vi "BonOMM-SAOMM.vi"() -> ()   [LabVIEW 2019] (continued)
                                n1515 = Bundle(w5154, w5153, "X"=w5137, "Y"=w5136) -> (w5155:cluster{void, void, "X":i32, "Y":i32})  [unwired: 1 in]
                                n1516 = property class="GraphInt (strict)"(reference=w5148, "Active Cursor"=u32 0) -> ("Y Scale.Range:Maximum"=w5139:dbl, "Y Scale.Range:Minimum"=w5138:dbl, "X Scale.Range:Maximum"=w5150:dbl, "X Scale.Range:Minimum"=w5149:dbl)  [unwired: 1 in, 2 out]
                                n1517 = call "BoxCrossPict.vi"("rect"=w5155) -> ("Pict Out"=→"Picture":picture)  [unwired: 1 in, 2 out]
                                n1518 = control-ref of="Picture"() -> (w5146:refnum<vi>)
                                n1519 = property class="Image"(reference=w5146) -> ("Draw Area Size"=w5147:T40)  [unwired: 1 in, 2 out]
                                n1520 = Unbundle(w5147) -> ("Width"=w5143:u32, "Height"=w5142:u32)
                                n1521 = Subtract(x=w5142, y=u32 6) -> (x-y=w5144:u32)
                                n1522 = Subtract(x=w5143, y=u32 6) -> (x-y=w5145:u32)
                                n1523 = call "Pict_to_Graph.vi"("Xo"=w5137, "Width"=w5145, "Yo"=w5136, "Heigth"=w5144, "X Scale.Range:Minimum"=w5149, "X Scale.Range:Maximum"=w5150, "Y Scale.Range:Minimum"=w5138, "Y Scale.Range:Maximum"=w5139) -> ()  [unwired: 2 in, 2 out]
                                }
                                frame True {
                                n1524 = property class="GraphInt (strict)"(reference=w5174, "Active Cursor"=u32 0) -> (reference out=w5166:refnum<vi>, "Y Scale.Range:Maximum"=w5170:dbl, "Y Scale.Range:Minimum"=w5169:dbl, "X Scale.Range:Maximum"=w5168:dbl, "X Scale.Range:Minimum"=w5167:dbl)  [unwired: 1 in, 1 out]
                                n1525 = control-ref of="Picture"() -> (w5163:refnum<vi>)
                                n1526 = property class="Image"(reference=w5163) -> ("Draw Area Size"=w5164:T40)  [unwired: 1 in, 2 out]
                                n1527 = Unbundle(w5164) -> ("Width"=w5162:u32, "Height"=w5161:u32)
                                n1528 = Subtract(x=w5161, y=u32 6) -> (x-y=w5157:u32)
                                n1529 = Subtract(x=w5162, y=u32 6) -> (x-y=w5158:u32)
                                n1530 = call "Pict_to_Graph.vi"("Xo"=w5175, "Width"=w5158, "Yo"=w5156, "Heigth"=w5157, "X Scale.Range:Minimum"=w5167, "X Scale.Range:Maximum"=w5168, "Y Scale.Range:Minimum"=w5169, "Y Scale.Range:Maximum"=w5170) -> ("CursorY"=w5172:dbl, "CursorX"=w5173:dbl)  [unwired: 2 in]
                                n1531 = property class="GraphInt (strict)"(reference=w5166, "Active Cursor"=u32 0, "Cursor.Cursor Position:Cursor X"=w5173, "Cursor.Cursor Position:Cursor Y"=w5172) -> ()  [unwired: 1 in, 2 out]
                                }
                                }
                              }
                            }
                            frame #1 {
                              n1532 = local read item#-1() -> (w5191)
                              n1533 = local read item#-1() -> (w5188)
                              n1534 = Max & Min(x=w5191, y=w5187) -> (min(x,y)=w5185:i32)  [unwired: 1 out]
                              n1535 = Max & Min(x=w5186, y=w5188) -> (max(x,y)=w5176:i32)  [unwired: 1 out]
                              n1536 = control-ref of="ImgArray"() -> (w5177:refnum<vi>)
                              n1537 = Subtract(x=w5191, y=w5187) -> (x-y=w5189:i32)
                              n1538 = Subtract(x=w5186, y=w5188) -> (x-y=w5190:i32)
                              n1539 = control-ref of="Picture"() -> (w5178:refnum<vi>)
                              n1540 = Absolute Value(x=w5189) -> (abs(x)=w5184:i32)
                              n1541 = Absolute Value(x=w5190) -> (abs(x)=w5183:i32)
                              n1542 = call "PICT_to_CAM.vi"("Pict Refnum"=w5178, "IntGraph Refnum"=w5177, "Ny"=w5183, "Yo"=w5176, "Nx"=w5184, "Xo"=w5185) -> ("Ny CAM"=→"Naxis2":i16, "Nx CAM"=→"Naxis1":i16, "Yo CAM"=w5181:i16, "Xo CAM"=w5182:i16)
                            }
                          }
                        }
                      }
                      n1543 = Not Equal?(x=w5115, y=w5117) -> (x != y?=w5118:bool)
                      n1544 = Not Equal?(x=w5117, y=w5114) -> (x != y?=w5119:bool)
                      n1545 = And(x=w5118, y=w5119) -> (x .and. y?=w5116:bool)
                    }
                  }
                  frame Enabled {
                  }
                }
              }
              event "TableXYPos": Cursor Grab {
                n1546 = event-data() -> ("CursIdx"=w5193:i32)  [unwired: 1 in, 7 out]
                n1547 = stacked-sequence {
                  tunnel: w5193 -> [w5194 _ _]
                  frame #0 {
                    n1548 = property on="TableXYPos" class="GraphXY (strict)"("Active Cursor"=w5194) -> ()  [unwired: 2 in, 2 out]
                    n1549 = case shown="1" w5194 {
                      tunnel: [TRUE FALSE] -> w5196
                      tunnel: [FALSE TRUE] -> w5195
                      frame 1 {
                      }
                      frame 0, Default {
                      }
                    }
                    n1550 = local write "act_cible"(w5195) -> ()
                    n1551 = local write "act_sonde"(w5196) -> ()
                  }
                  frame #1 {
                    n1552 = local read "ImgData"() -> (w5201:sgl[][])
                    n1553 = while {
                      tunnel: w5201 -> [w5204]
                      stop <- w5202 stop-if-true
                      n1554 = event shown="[0] Timeout" {
                        selector: _ -> [_ _]
                        dyn-events: _ -> [_ _]
                        timeout: 100 -> [_ _]
                        tunnel: w5204 -> [_ _]
                        tunnel: [FALSE TRUE] -> w5202
                        event Timeout {
                          w5205 = u16 1 items=["Region d'intérêt", "Prévisualisation"] ("ImageUsage")
                          n1555 = event-data() -> ()  [unwired: 1 in, 2 out]
                          n1556 = property on="TableXYPos" class="GraphXY (strict)"("Active Cursor"=u32 0) -> (error out=w5209:errorcluster)  [unwired: 2 in, 1 out]
                          n1557 = property on="TableXYPos" class="GraphXY (strict)"(error in=w5209) -> ("Cursor.Cursor X"=w5217:dbl, "Cursor.Cursor Y"=w5216:dbl)  [unwired: 1 in, 2 out]
                          n1558 = local read "FieldAstrom"() -> (w5211:T4)
                          n1559 = call "xy2ad.vi"("Y (px)"=w5216, "X (px)"=w5217, "Astrometry"=w5211) -> ("DEC (°)"=w5213:dbl, "RA (°)"=w5214:dbl, "DEC (HH:MM:SS)"=w5215:dbl, "RA (HH:MM:SS.S)"=w5212:dbl)  [unwired: 5 in]
                          n1560 = local read "ImgAstrom"() -> (w5225:T4)
                          n1561 = local write "RA Cible"(w5212) -> ()
                          n1562 = local write "Dec Cible"(w5215) -> ()
                          n1563 = local read "ImgData"() -> (w5218:sgl[][])
                          n1564 = call "ad2xy.vi"("DEC"=w5213, "RA"=w5214, "Astrometry"=w5225) -> ("Y"=w5224:dbl, "X"=w5223:dbl)  [unwired: 6 in, 1 out]
                          n1565 = To Long Integer(number=w5223) -> (32bit integer=w5220:i32)
                          n1566 = To Long Integer(number=w5224) -> (32bit integer=w5219:i32)
                          n1567 = call "subimage.vi"("Ysz/2"=100 ("Xsz/2"), "Xsz/2"=100, "Yc"=w5219, "Xc"=w5220, "ImgData"=w5218) -> ("SubImg"=w5207:sgl[][])  [unwired: 6 in]
                          n1568 = Array Max & Min(array=w5207) -> (max value=w5206:sgl)  [unwired: 3 out]
                          n1569 = call "Draw_crosshair.vi"("Image IN"=w5207, "White Value"=w5206) -> ("Image OUT"=→"subimg":sgl[][])  [unwired: 13 in]
                          n1570 = local write "ImageUsage"(w5205) -> ()
                        }
                        event "TableXYPos": Cursor Release {
                          n1571 = event-data() -> ()  [unwired: 1 in, 8 out]
                        }
                      }
                    }
                  }
                  frame #2 {
                    n1572 = local write "CursorGrab"(FALSE ("CursorGrab")) -> ()
                  }
                }
                "CursorGrab" <- TRUE ("CursorGrab")
              }
              event "RA Cible", "Dec Cible", "RA Sonde", "Dec Sonde", "act_cible", "act_sonde": Mouse Down {
                n1573 = event-data() -> ("CtlRef"=w5232:refnum<vi>)  [unwired: 1 in, 6 out]
                n1574 = property class="Cmde"(reference=w5232) -> ("Label.Text"=w5231:string)  [unwired: 1 in, 2 out]
                n1575 = case shown="\"Dec Cible\", \"RA Cible\", \"act_cible\", Par défaut" w5231 {
                  tunnel: [TRUE FALSE] -> w5229
                  tunnel: [FALSE TRUE] -> w5230
                  frame "Dec Sonde", "RA Sonde", "act_sonde" {
                  }
                  frame "Dec Cible", "RA Cible", "act_cible", Default {
                  }
                }
                "act_sonde" <- w5229
                "act_cible" <- w5230
              }
              event "N.O. A.D.", "N.O. Déc.", "NO epoch": Value Change {
                # "Peut-être qu'ici on"
                n1576 = event-data() -> ()  [unwired: 1 in, 6 out]
                n1577 = local read "N.O. Déc."() -> (w5250:string)
                n1578 = local read "N.O. A.D."() -> (w5251:string)
                n1579 = call "format_coords_str(new).vi"("DEC str"=w5250, "RA str"=w5251) -> ("%s DEC"=w5248:string, "%s RA"=w5249:string)  [unwired: 1 in]
                n1580 = local read "NO epoch"() -> (w5247:dbl)
                n1581 = call "time-str-to-time-dbl-RA.vi"("Chaîne"=w5249) -> ("TCS_coords"=w5240:dbl)
                n1582 = call "time-str-to-time-dbl-DEC.vi"("Chaîne"=w5248) -> ("TCS_coords"=w5238:dbl)
                n1583 = local read "LST"() -> (w5246:dbl)
                n1584 = expression code="x*3600"(w5240) -> (w5239:dbl)
                n1585 = expression code="x*3600"(w5238) -> (w5237:dbl)
                n1586 = call "Object_properties.vi"("Target RA"=w5239, "Target DEC"=w5237, "Target Epoch"=w5247, "Sideral Time"=w5246) -> ("NO RA"=w5245:string, "NO DEC"=w5244:string, "NO Epoch"=w5242:dbl, "NO HA"=w5241:dbl, "NO AM"=w5243:dbl)  [unwired: 7 in]
                n1587 = local write "NO AM"(w5243) -> ()
                n1588 = local write "NO HA"(w5241) -> ()
                n1589 = local write "NO epoch"(w5242) -> ()
                n1590 = local write "N.O. Déc."(w5244) -> ()
                n1591 = local write "N.O. A.D."(w5245) -> ()
              }
              event "Flat": Value Change {
                n1592 = event-data() -> ("NewVal"=w5255:bool)  [unwired: 1 in, 4 out]
                n1593 = Select(t="Ouverture" ("Indicateur d'état"), s=w5255, f="Fermeture" ("Indicateur d'état")) -> (s? t:f=w5259:string)
                n1594 = local read "Calib VRN"() -> (w5263:refnum<visa-resource-name>)
                n1595 = Concatenate Strings(w5259, " de la lampe de flat" ("Indicateur d'état")) -> (w5262:string)
                n1596 = control-ref of="TERMINAL"() -> (w5256:refnum<vi>)
                n1597 = control-ref of="Indicateur d'état"() -> (w5257:refnum<vi>)
                n1598 = Build Array("Arc", "Néon", w5255) -> (w5264:bool[])
                n1599 = call "Controle_des_lampe.vi"("VISA resource name"=w5263, "Status In"=w5264) -> ("Status Out"=w5254:bool[])  [unwired: 2 out]
                n1600 = local write "Status lamp"(w5254) -> ()
                n1601 = call "TERMINAL.vi"("Indicateur Refnum"=w5257, "Terminal Refnum"=w5256, "Indicateur d'état"=w5262) -> ()
                n1602 = Index Array(array=w5254, index=0 ("Index")) -> (element=→"ArcOn":bool)
                n1603 = Index Array(array=w5254, index=1 ("Index")) -> (element=→"NeonOn":bool)
                n1604 = Index Array(array=w5254, index=2 ("Index")) -> (element=→"FlatOn":bool)
                n1605 = Boolean Array To Number(Boolean array=w5254) -> (number=w5253:u32)
                n1606 = Greater Than 0?(x=w5253) -> (x > 0?=w5252:bool)
                n1607 = property on="lampOn?" class="Bool (strict)"("Blinking"=w5252, "Visible"=w5252) -> ()  [unwired: 2 in, 2 out]
              }
              event "Néon": Value Change {
                n1608 = event-data() -> ("NewVal"=w5276:bool)  [unwired: 1 in, 4 out]
                n1609 = local read "Arc"() -> (w5293:bool)
                n1610 = Select(t="Ouverture" ("Indicateur d'état"), s=w5276, f="Fermeture" ("Indicateur d'état")) -> (s? t:f=w5280:string)
                n1611 = Build Array(w5293, w5276, "Flat") -> (w5286:bool[])
                n1612 = local read "Calib VRN"() -> (w5284:refnum<visa-resource-name>)
                n1613 = Concatenate Strings(w5280, " de la lampe de Néon" ("Indicateur d'état")) -> (w5277:string)
                n1614 = call "Controle_des_lampe.vi"("VISA resource name"=w5284, "Status In"=w5286) -> ("Status Out"=w5273:bool[])  [unwired: 2 out]
                n1615 = local write "Status lamp"(w5273) -> ()
                n1616 = control-ref of="TERMINAL"() -> (w5283:refnum<vi>)
                n1617 = control-ref of="Indicateur d'état"() -> (w5282:refnum<vi>)
                n1618 = call "TERMINAL.vi"("Indicateur Refnum"=w5282, "Terminal Refnum"=w5283, "Indicateur d'état"=w5277) -> ()
                n1619 = Boolean Array To Number(Boolean array=w5273) -> (number=w5274:u32)
                n1620 = Index Array(array=w5273, index=0 ("Index")) -> (element=w5290:bool)
                n1621 = Index Array(array=w5273, index=1 ("Index")) -> (element=w5291:bool)
                n1622 = Index Array(array=w5273, index=2 ("Index")) -> (element=w5292:bool)
                n1623 = Greater Than 0?(x=w5274) -> (x > 0?=w5275:bool)
                n1624 = local write "NeonOn"(w5291) -> ()
                n1625 = local write "ArcOn"(w5290) -> ()
                n1626 = local write "FlatOn"(w5292) -> ()
                n1627 = property on="lampOn?" class="Bool (strict)"("Blinking"=w5275, "Visible"=w5275) -> ()  [unwired: 2 in, 2 out]
              }
              event "Arc": Value Change {
                n1628 = event-data() -> ("NewVal"=w5297:bool)  [unwired: 1 in, 4 out]
                n1629 = local read "Néon"() -> (w5314:bool)
                n1630 = local read "Flat"() -> (w5306:bool)
                n1631 = Select(t="Ouverture" ("Indicateur d'état"), s=w5297, f="Fermeture" ("Indicateur d'état")) -> (s? t:f=w5301:string)
                n1632 = Build Array(w5297, w5314, w5306) -> (w5307:bool[])
                n1633 = local read "Calib VRN"() -> (w5305:refnum<visa-resource-name>)
                n1634 = call "Controle_des_lampe.vi"("VISA resource name"=w5305, "Status In"=w5307) -> ("Status Out"=w5294:bool[])  [unwired: 2 out]
                n1635 = local write "Status lamp"(w5294) -> ()
                n1636 = Concatenate Strings(w5301, " de la lampe à arc" ("Indicateur d'état")) -> (w5298:string)
                n1637 = control-ref of="TERMINAL"() -> (w5304:refnum<vi>)
                n1638 = control-ref of="Indicateur d'état"() -> (w5303:refnum<vi>)
                n1639 = Index Array(array=w5294, index=0 ("Index")) -> (element=w5311:bool)
                n1640 = Index Array(array=w5294, index=1 ("Index")) -> (element=w5312:bool)
                n1641 = Index Array(array=w5294, index=2 ("Index")) -> (element=w5313:bool)
                n1642 = Boolean Array To Number(Boolean array=w5294) -> (number=w5296:u32)
                n1643 = call "TERMINAL.vi"("Indicateur Refnum"=w5303, "Terminal Refnum"=w5304, "Indicateur d'état"=w5298) -> ()
                n1644 = Greater Than 0?(x=w5296) -> (x > 0?=w5295:bool)
                n1645 = local write "NeonOn"(w5312) -> ()
                n1646 = local write "ArcOn"(w5311) -> ()
                n1647 = local write "FlatOn"(w5313) -> ()
                n1648 = property on="lampOn?" class="Bool (strict)"("Blinking"=w5295, "Visible"=w5295) -> ()  [unwired: 2 in, 2 out]
              }
              event "ModCoor": Value Change {
                n1649 = event-data() -> ("NewVal"=w5316:bool)  [unwired: 1 in, 4 out]
                n1650 = case shown="Vrai" w5316 {
                  tunnel: [FALSE w5319] -> w5315
                  frame False {
                  }
                  frame True {
                    # "Système acquisition ou\ntechnicien est prioritaire"
                    # "Epoque=0=>courante du TCS"
                    n1651 = call "time-str-to-time-dbl-DEC.vi"("Chaîne"="N.O. Déc.") -> ("TCS_coords"=w5328:dbl)
                    n1652 = call "time-str-to-time-dbl-RA.vi"("Chaîne"="N.O. A.D.") -> ("TCS_coords"=w5327:dbl)
                    n1653 = control-ref of="TERMINAL"() -> (w5335:refnum<vi>)
                    n1654 = control-ref of="Indicateur d'état"() -> (w5336:refnum<vi>)
                    n1655 = control-ref of="TCS actif"() -> (w5320:refnum<vi>)
                    n1656 = Concatenate Strings("Chargement des coordonnées : ", "N.O. A.D.", ", ", "N.O. Déc.") -> (w5330:string)
                    n1657 = local read "TCS VRN"() -> (w5325:refnum<visa-resource-name>)
                    n1658 = Build Array(w5327, w5328, "NO epoch") -> (w5326:dbl[])
                    n1659 = call "TERMINAL.vi"("Indicateur Refnum"=w5336, "Terminal Refnum"=w5335, "Indicateur d'état"=w5330) -> ()
                    n1660 = call "EXCOM-CMD.vi"("VRN IN"=w5325, "Bool Refnum"=w5320, "Commande #"=6, "Args"=w5326) -> ("VRN OUT"=w5321:refnum<visa-resource-name>, "OK Done"=w5323:bool, "Error OUT"=w5322:errorcluster)  [unwired: 9 in]
                    n1661 = local write "ModCoor"(FALSE) -> ()
                    n1662 = local write "TCS Error"(w5322) -> ()
                    n1663 = local write "TCS VRN"(w5321) -> ()
                    n1664 = case shown="Vrai" w5323 {
                      tunnel: [FALSE w5341] -> w5319
                      frame False {
                        n1665 = One Button Dialog(message="ATTENTION!!\nProblème d'écriture\ndes nouvelles coordonnées.\nVérifiez TCS.", button name ("OK")="OK" ("nom du bouton (\"OK\")")) -> ()  [unwired: 1 out]
                      }
                      frame True {
                        w5341 = TRUE
                        n1666 = local read "STATL"() -> (w5342:bool[])
                        n1667 = Index Array(array=w5342, index=2 ("Index")) -> ()  [unwired: 1 out]
                        n1668 = case shown="Faux" w5341 {
                          frame False {
                            n1669 = One Button Dialog(message="ATTENTION!!\nLe télescope n'est pas en \nMODE ENTRAÎNEMENT SIDÉRAL.", button name ("OK")="OK" ("nom du bouton (\"OK\")")) -> ()  [unwired: 1 out]
                          }
                          frame True {
                          }
                        }
                      }
                    }
                  }
                }
                n1670 = case shown="Vrai" w5315 {
                  frame False {
                  }
                  frame True {
                    n1671 = property on="GO" class="Bool (strict)"("Key Focus"=TRUE) -> ()  [unwired: 2 in, 2 out]
                  }
                }
              }
              event "SaveCoords": Value Change {
                n1672 = event-data() -> ()  [unwired: 1 in, 5 out]
                n1673 = flat-sequence {
                  tunnel: [w5353] -> w5349
                  tunnel: [w5352] -> w5348
                  tunnel: [w5351] -> w5347
                  tunnel: [w5350] -> w5346
                  tunnel: w5349 -> [w5359]
                  tunnel: w5348 -> [w5360]
                  tunnel: w5347 -> [w5361]
                  tunnel: w5346 -> [w5358]
                  frame #0 {
                    n1674 = local read "Epoch Tel"() -> (w5354:dbl)
                    n1675 = local read "DEC Tel"() -> (w5356:dbl)
                    n1676 = local read "RA Tel"() -> (w5355:dbl)
                    n1677 = local write "SaveCoords"(FALSE ("SaveCoords")) -> ()
                    n1678 = call "SaveCoords.vi"("Epoch Tel"=w5354, "DEC Tel"=w5356, "RA Tel"=w5355) -> ("Accepted?"=w5350:bool, "Epoch Out"=w5351:dbl, "DEC Out"=w5352:dbl, "RA Out"=w5353:dbl)  [unwired: 5 in]
                  }
                  frame #1 {
                    n1679 = case shown="Vrai" w5358 {
                      tunnel: w5361 -> [_ w5365]
                      tunnel: w5360 -> [_ w5364]
                      tunnel: w5359 -> [_ w5363]
                      frame False {
                      }
                      frame True {
                        w5389 = "\t"
                        w5382 = "_"
                        w5376 = TRUE ("replace all? (F)")
                        w5375 = " "
                        w5374 = "0"
                        w5371 = i16 2 ("width (-)")
                        w5370 = i16 0 ("width (-)")
                        n1680 = call "time-sec-to-time-str-DEC.vi"("Numeric"=w5363) -> ("formatted-str"=w5386:string)
                        n1681 = call "time-sec-to-time-str-DEC.vi"("Numeric"=w5364) -> ("formatted-str"=w5387:string)
                        n1682 = Number To Fractional String(number=w5365, width (-)=i16 4, precision (6)=i16 2) -> (F-format string=w5388:string)  [unwired: 1 in]
                        n1683 = Get Date/Time String() -> (time string=w5385:string)  [unwired: 3 in, 1 out]
                        n1684 = local read "From library"() -> (w5366:bool)
                        n1685 = Concatenate Strings(w5385, w5389, w5386, w5389, w5387, w5389, w5388, "\r\n") -> (w5391:string)
                        n1686 = call "GetUTC.vi"() -> ("Day"=w5396:dbl, "Month"=w5395:dbl, "Year"=w5394:dbl)  [unwired: 6 out]
                        n1687 = case shown="Vrai" w5366 {
                          tunnel: [FALSE FALSE] -> w5362
                          tunnel: w5386 -> [w5400 w5407]
                          tunnel: w5387 -> [w5399 w5408]
                          tunnel: w5388 -> [w5398 w5409]
                          tunnel: w5385 -> [w5397 w5406]
                          frame False {
                            w5402 = i16 0 items=["tel coords", "tel offset", "guidage"] ("options")
                            n1688 = local read "Obslib"() -> (w5403:string[][])
                            n1689 = Build Array(w5400, w5399, w5398, w5397) -> (w5404:string[])
                            n1690 = call "Coords to chart(new).vi"("DataLine"=w5404, "options"=w5402, "Tableau entrant"=w5403) -> ("historique"=w5405:string[][])
                            n1691 = local write "Obslib"(w5405) -> ()
                          }
                          frame True {
                            w5411 = i16 0 items=["tel coords", "tel offset", "guidage"] ("options")
                            n1692 = local read "Obslib"() -> (w5412:string[][])
                            n1693 = Build Array(w5407, w5408, w5409, w5406) -> (w5413:string[])
                            n1694 = call "Coords to chart(new).vi"("DataLine"=w5413, "options"=w5411, "Tableau entrant"=w5412) -> ("historique"=w5414:string[][])
                            n1695 = local write "Obslib"(w5414) -> ()
                          }
                        }
                        n1696 = Number To Fractional String(number=w5394, width (-)=i16 4, precision (6)=w5370) -> (F-format string=w5377:string)  [unwired: 1 in]
                        n1697 = Number To Fractional String(number=w5395, width (-)=w5371, precision (6)=w5370) -> (F-format string=w5372:string)  [unwired: 1 in]
                        n1698 = Number To Fractional String(number=w5396, width (-)=w5371, precision (6)=w5370) -> (F-format string=w5373:string)  [unwired: 1 in]
                        n1699 = Search and Replace String(replace all?=w5376, input string=w5372, search string=w5375, replace string=w5374) -> (result string=w5378:string)  [unwired: 4 in, 3 out]
                        n1700 = Search and Replace String(replace all?=w5376, input string=w5373, search string=w5375, replace string=w5374) -> (result string=w5379:string)  [unwired: 4 in, 3 out]
                        n1701 = local read "path_pointing"() -> (w5380:path)
                        n1702 = Concatenate Strings(w5377, w5382, w5378, w5382, w5379, ".pnt") -> (w5381:string)
                        n1703 = Build Path(base path=w5380, name or relative path=w5381) -> (appended path=w5384:path)
                        n1704 = local read "File I/O Error"() -> (w5393:errorcluster)
                        n1705 = Write to Text File(file (use dialog)=w5384, text=w5391, error in=w5393) -> (error out=w5392:errorcluster)  [unwired: 1 in, 2 out]
                        n1706 = local write "From library"(w5362) -> ()
                        n1707 = local write "File I/O Error"(w5392) -> ()
                      }
                    }
                  }
                }
              }
              event "NO RA clic-sim": Value Change; "N.O. A.D.": Mouse Down {
                n1708 = event-data() -> ()  [unwired: 1 in, 4 out]
                n1709 = local write "N.O. A.D."("") -> ()
                n1710 = local write "NO epoch"(2000.0 ("NO epoch")) -> ()
                "NO RA clic-sim" <- FALSE
              }
              event "N.O. Déc.": Mouse Down {
                n1711 = event-data() -> ()  [unwired: 1 in, 8 out]
                n1712 = local write "NO epoch"(2000.0 ("NO epoch")) -> ()
                n1713 = local write "N.O. Déc."("") -> ()
              }
              event "Zénith", "Écran", "Range": Value Change {
                n1714 = event-data() -> ()  [unwired: 1 in, 1 out]
                n1715 = local read "Mode Est"() -> (w5420:bool)
                n1716 = case shown="Faux" w5420 {
                  selector: w5420 -> [_ w5635]
                  frame False {
                    # "Track ON ou OFF"
                    n1717 = local read "STATL"() -> (w5425:bool[])
                    n1718 = Index Array(array=w5425, index=2 ("Index")) -> (element=w5424:bool)
                    n1719 = case shown="Faux" w5424 {
                      tunnel: "Range" -> [w5430 _]
                      tunnel: "Zénith" -> [w5429 _]
                      tunnel: "Écran" -> [w5428 _]
                      frame False {
                        w5427 = FALSE
                        w5433 = string[] ["RANGEMENT", "ZÉNITH", "ÉCRAN"]
                        w5438 = 0
                        n1720 = local read "TCS VRN"() -> (w5437:refnum<visa-resource-name>)
                        n1721 = control-ref of="TERMINAL"() -> (w5435:refnum<vi>)
                        n1722 = control-ref of="Indicateur d'état"() -> (w5436:refnum<vi>)
                        n1723 = Select(t=1, s=w5430, f=w5438) -> (s? t:f=w5446:i32)
                        n1724 = Select(t=2, s=w5429, f=w5438) -> (s? t:f=w5444:i32)
                        n1725 = Select(t=3, s=w5428, f=w5438) -> (s? t:f=w5445:i32)
                        n1726 = Compound Arithmetic op=ADD(w5446, w5444, w5445) -> (w5443:i32)
                        n1727 = local write "Zénith"(w5427) -> ()
                        n1728 = local write "Écran"(w5427) -> ()
                        n1729 = local write "Range"(w5427) -> ()
                        n1730 = Decrement(x=w5443) -> (x-1=w5434:i32)
                        n1731 = Index String Array(1:w5434, 2:w5433, 3:"Le télescope va se déplacer\nvers la position ") -> (0:w5442:string)
                        n1732 = Two Button Dialog(message=w5442, 1:"Annulez" ("Nom du bouton F (\"Annuler\")"), 2:"OK" ("Nom du bouton V (\"OK\")")) -> (T button?=w5450:bool)
                        n1733 = Index String Array(1:w5434, 2:w5433, 3:"Commande de déplacement : " ("string (\"\")")) -> (0:w5431:string)
                        n1734 = call "TERMINAL.vi"("Indicateur Refnum"=w5436, "Terminal Refnum"=w5435, "Indicateur d'état"=w5431) -> ()
                        n1735 = case shown="Vrai" w5450 {
                          selector: w5450 -> [w5451 _]
                          tunnel: w5434 -> [_ w5455]
                          tunnel: w5430 -> [_ w5454]
                          tunnel: w5433 -> [_ w5453]
                          tunnel: w5437 -> [_ w5452]
                          frame False {
                            n1736 = local write "Zénith"(w5451) -> ()
                            n1737 = local write "Écran"(w5451) -> ()
                            n1738 = local write "Range"(w5451) -> ()
                          }
                          frame True {
                            n1739 = stacked-sequence {
                              seq-local: [w5457 _ _] -> [_ _ w5627]
                              tunnel: w5455 -> [w5458 w5486 _]
                              tunnel: w5454 -> [_ w5493 _]
                              tunnel: w5453 -> [_ w5492 _]
                              tunnel: w5452 -> [w5456 w5491 _]
                              frame #0 {
                                n1740 = disable-structure shown="Disabled" {
                                disable-tunnel: [w5460 _] -> w5457
                                disable-tunnel: w5456 -> [w5459 _]
                                frame Disabled {
                                n1741 = flat-sequence {
                                tunnel: [w5462] -> w5460
                                tunnel: w5459 -> [w5466]
                                tunnel: [w5464] -> w5461
                                tunnel: w5461 -> [w5469]
                                frame #0 {
                                n1742 = local read "Epoch Tel"() -> (w5463:dbl)
                                n1743 = Build Array(w5463) -> (w5462:dbl[])
                                }
                                frame #1 {
                                n1744 = local read "AnnéeRL"() -> (w5464:dbl)
                                n1745 = control-ref of="TCS actif"() -> (w5465:refnum<vi>)
                                n1746 = Build Array(w5464) -> (w5468:dbl[])
                                n1747 = call "EXCOM-CMD.vi"("VRN IN"=w5466, "Bool Refnum"=w5465, "Commande #"=22, "Args"=w5468) -> ()  [unwired: 9 in, 3 out]
                                }
                                frame #2 {
                                n1748 = while {
                                tunnel: [w5472] -> _
                                tunnel: w5469 -> [w5470]
                                i -> [w5479]
                                stop <- w5476 stop-if-true
                                # "Environ 1 jour ..."
                                n1749 = local read "Epoch Tel"() -> (w5475:dbl)
                                n1750 = Subtract(x=w5475, y=w5470) -> (x-y=w5474:dbl)
                                n1751 = Absolute Value(x=w5474) -> (abs(x)=w5473:dbl)
                                n1752 = Less Or Equal?(x=w5473, y=0.002) -> (x <= y?=w5472:bool)
                                n1753 = call "Max-iteration.vi"("i max"=500, "i act"=w5479, "Valeur entrante"=w5472) -> ("break ?"=w5476:bool)
                                n1754 = Wait (ms)(milliseconds to wait=u32 10) -> ()  [unwired: 1 out]
                                }
                                }
                                }
                                }
                                frame Enabled {
                                }
                                }
                                n1755 = disable-structure shown="Disabled" {
                                disable-tunnel: w5458 -> [w5480 _]
                                frame Disabled {
                                n1756 = case shown="2" w5480 {
                                frame 0, Default {
                                n1757 = property on="Range" class="Bool (strict)"("Blinking"=TRUE) -> ()  [unwired: 2 in, 2 out]
                                }
                                frame 1 {
                                n1758 = property on="Zénith" class="Bool (strict)"("Blinking"=TRUE) -> ()  [unwired: 2 in, 2 out]
                                }
                                frame 2 {
                                n1759 = property on="Écran" class="Bool (strict)"("Blinking"=TRUE) -> ()  [unwired: 2 in, 2 out]
                                }
                                }
                                }
                                frame Enabled {
                                }
                                }
                              }
                              frame #1 {
                                n1760 = case shown="2" w5486 {
                                selector: w5486 -> [w5596 w5600 w5604]
                                tunnel: [w5596 w5600 w5604] -> w5485
                                tunnel: [w5599 w5603 w5607] -> w5484
                                frame 0, Default {
                                n1761 = Build Array(4.0 ("element"), 10.0 ("element")) -> (w5599:dbl[])
                                }
                                frame 1 {
                                n1762 = Build Array(0.0 ("element"), 45.45556 ("element")) -> (w5603:dbl[])
                                }
                                frame 2 {
                                n1763 = Build Array(5.0 ("element"), 56.0 ("element")) -> (w5607:dbl[])
                                }
                                }
                                n1764 = property on="Position Z" class="NumNb (strict)" props=["Value"]() -> ()  [unwired: 2 in, 3 out]
                                n1765 = control-ref of="TCS actif"() -> (w5487:refnum<vi>)
                                n1766 = case shown="Vrai" w5493 {
                                frame False {
                                }
                                frame True {
                                n1767 = Two Button Dialog(message="Ranger la sonde aussi?", 1:"Non" ("F button name (\"Cancel\")"), 2:"Oui" ("T button name (\"OK\")")) -> (T button?=w5608:bool)
                                n1768 = case shown="Vrai" w5608 {
                                frame False {
                                }
                                frame True {
                                n1769 = local read "Table VRN"() -> (w5623:refnum<visa-resource-name>)
                                n1770 = local read "Table Error"() -> (w5615:errorcluster)
                                n1771 = local read "Rangement Y"() -> (w5619:dbl)
                                n1772 = local read "Rangement X"() -> (w5620:dbl)
                                n1773 = local read "Rangement Z"() -> (w5618:dbl)
                                n1774 = local read "BrasPesto"() -> (w5612:bool)
                                n1775 = local read "LimXPesto"() -> (w5613:dbl)
                                n1776 = control-ref of="Table actif"() -> (w5624:refnum<vi>)
                                n1777 = call "Newmark-GotoAll.vi"("Table VRN IN"=w5623, "BrasPesto"=w5612, "Bool Refnum"=w5624, "LimXPesto"=w5613, "Notify?"=FALSE, "Error IN"=w5615, "Position X"=w5620, "Position Y"=w5619, "Position Z"=w5618) -> ("Table VRN OUT"=w5622:refnum<visa-resource-name>, "Error OUT"=w5614:errorcluster)  [unwired: 5 in]
                                n1778 = Unbundle By Name(w5614) -> ("status"=w5617:bool)
                                n1779 = local write "Table Error"(w5614) -> ()
                                n1780 = local write "Table VRN"(w5622) -> ()
                                n1781 = Not(x=w5617) -> (.not. x?=w5616:bool)
                                n1782 = case shown="Vrai" w5616 {
                                frame False {
                                n1783 = One Button Dialog(message="ATTENTION!!\nLa commande RangeTable a échoué.\nVérifiez le contrôleur des tables.", button name ("OK")="OK" ("nom du bouton (\"OK\")")) -> ()  [unwired: 1 out]
                                }
                                frame True {
                                }
                                }
                                }
                                }
                                }
                                }
                                n1784 = call "EXCOM-CMD.vi"("VRN IN"=w5491, "Bool Refnum"=w5487, "Commande #"=36, "Args"=w5484) -> ("VRN OUT"=w5489:refnum<visa-resource-name>, "OK Done"=w5494:bool, "Error OUT"=w5488:errorcluster)  [unwired: 9 in]
                                n1785 = case shown="Vrai" w5494 {
                                tunnel: w5492 -> [w5499 _]
                                tunnel: w5485 -> [w5498 w5522]
                                tunnel: w5489 -> [w5497 w5517]
                                tunnel: w5488 -> [w5496 w5516]
                                tunnel: w5487 -> [w5495 w5514]
                                frame False {
                                n1786 = Index String Array(1:w5498, 2:w5499, 3:"ATTENTION!!\nLa commande" ("chaîne (\"\")")) -> (0:w5503:string)
                                n1787 = Concatenate Strings(w5503, " a échoué.\nAnnulez la commande." ("chaîne")) -> (w5500:string)
                                n1788 = One Button Dialog(message=w5500, button name ("OK")="OK" ("nom du bouton (\"OK\")")) -> (true=w5504:bool)
                                n1789 = case shown="Vrai" w5504 {
                                tunnel: w5497 -> [_ w5510]
                                tunnel: w5496 -> [_ w5509]
                                tunnel: w5495 -> [_ w5506]
                                frame False {
                                }
                                frame True {
                                n1790 = call "EXCOM-CMD.vi"("VRN IN"=w5510, "Bool Refnum"=w5506, "Commande #"=13, "Error IN"=w5509) -> ("OK Done"=w5507:bool)  [unwired: 9 in, 2 out]
                                n1791 = case shown="Faux" w5507 {
                                frame False {
                                n1792 = One Button Dialog(message="ATTENTION!!\nLa commande STOP a échoué.\nVérifiez TCS.", button name ("OK")="OK" ("nom du bouton (\"OK\")")) -> ()  [unwired: 1 out]
                                }
                                frame True {
                                n1793 = Wait (ms)(milliseconds to wait=u32 10 ("attente (ms)")) -> ()  [unwired: 1 out]
                                }
                                }
                                }
                                }
                                }
                                frame True {
                                # "Est-ce qu'ici on pourrait utiliser\nl'information déjà obtenue ?"
                                # "Drives ON ?"
                                n1794 = call "EXCOM-26.vi"("VRN IN"=w5517, "Bool Refnum"=w5514, "Error IN"=w5516) -> ("STATH"=w5519:bool[], "VRN OUT"=w5518:refnum<visa-resource-name>, "Error OUT"=w5515:errorcluster)  [unwired: 6 in, 4 out]
                                n1795 = Index Array(array=w5519, index=7 ("Index")) -> (element=w5520:bool)
                                n1796 = case shown="Vrai" w5520 {
                                tunnel: w5522 -> [_ w5547]
                                tunnel: w5518 -> [w5527 w5546]
                                tunnel: w5515 -> [w5526 w5545]
                                tunnel: [w5523 w5544] -> _
                                tunnel: [w5525 w5543] -> _
                                tunnel: [w5524 w5542] -> _
                                tunnel: w5514 -> [_ w5541]
                                frame False {
                                n1797 = stacked-sequence {
                                tunnel: w5527 -> [_ w5535 _]
                                tunnel: w5526 -> [_ w5533 _]
                                tunnel: [_ w5532 _] -> w5523
                                tunnel: [_ w5531 _] -> w5525
                                tunnel: [_ w5530 _] -> w5524
                                frame #0 {
                                n1798 = One Button Dialog(message="ATTENTION!!\nLes moteurs ne sont pas allumés. ", button name ("OK")="OK" ("nom du bouton (\"OK\")")) -> ()  [unwired: 1 out]
                                }
                                frame #1 {
                                n1799 = call "EXCOM-CMD.vi"("VRN IN"=w5535, "Commande #"=13, "Error IN"=w5533) -> ("VRN OUT"=w5531:refnum<visa-resource-name>, "OK Done"=w5530:bool, "Error OUT"=w5532:errorcluster)  [unwired: 10 in]
                                n1800 = case shown="Faux" w5530 {
                                frame False {
                                n1801 = One Button Dialog(message="ATTENTION!!\nLa commande STOP a échoué.\nVérifiez TCS.", button name ("OK")="OK" ("nom du bouton (\"OK\")")) -> ()  [unwired: 1 out]
                                }
                                frame True {
                                n1802 = Wait (ms)(milliseconds to wait=u32 10 ("attente (ms)")) -> ()  [unwired: 1 out]
                                }
                                }
                                }
                                frame #2 {
                                w5539 = 0
                                w5540 = FALSE ("Blinking")
                                n1803 = property on="Zénith" class="Bool (strict)"("Disabled"=w5539) -> ()  [unwired: 2 in, 2 out]
                                n1804 = property on="Range" class="Bool (strict)"("Disabled"=w5539) -> ()  [unwired: 2 in, 2 out]
                                n1805 = property on="Écran" class="Bool (strict)"("Disabled"=w5539) -> ()  [unwired: 2 in, 2 out]
                                n1806 = property on="Zénith" class="Bool (strict)"("Blinking"=w5540) -> ()  [unwired: 2 in, 2 out]
                                n1807 = property on="Range" class="Bool (strict)"("Blinking"=w5540) -> ()  [unwired: 2 in, 2 out]
                                n1808 = property on="Écran" class="Bool (strict)"("Blinking"=w5540) -> ()  [unwired: 2 in, 2 out]
                                }
                                }
                                }
                                frame True {
                                n1809 = stacked-sequence {
                                tunnel: w5547 -> [w5562 _]
                                tunnel: w5546 -> [w5561 w5593]
                                tunnel: w5545 -> [_ w5591]
                                tunnel: [_ w5590] -> w5544
                                tunnel: [_ w5589] -> w5543
                                tunnel: [_ w5588] -> w5542
                                tunnel: w5541 -> [w5549 w5587]
                                frame #0 {
                                # "Est-ce qu'ici on pourrait utiliser\nl'information déjà obtenue ?"
                                n1810 = local read "dflt-EQX"() -> (w5548:dbl)
                                n1811 = call "EXCOM-25-EQ.vi"("VISA resource name"=w5561, "Bool Refnum"=w5549, "Display Equinox"=w5548) -> ("RA"=w5556:dbl, "DEC"=w5555:dbl, "Epoque"=w5550:dbl, "Temps Sidéral"=w5551:dbl)  [unwired: 2 in, 11 out]
                                n1812 = case shown="0" w5562 {
                                tunnel: w5551 -> [w5565 w5574 w5580 _]
                                tunnel: [w5564 w5574 w5576 w5586] -> w5558
                                tunnel: [36000.0 ("y") 163640.0 ("Nouvelle Déc.") 201600.0 ("Nouvelle Déc.") w5585] -> w5557
                                tunnel: w5556 -> [_ _ _ w5586]
                                tunnel: w5555 -> [_ _ _ w5585]
                                frame 0 {
                                n1813 = Subtract(x=w5565, y=14400.0) -> (x-y=w5566:dbl)
                                n1814 = Less Than 0?(x=w5566) -> (x < 0?=w5567:bool)
                                n1815 = case shown="Vrai" w5567 {
                                tunnel: w5566 -> [w5569 w5571]
                                tunnel: [w5569 w5570] -> w5564
                                frame False {
                                }
                                frame True {
                                n1816 = Add(x=w5571, y=86400.0) -> (x+y=w5570:dbl)
                                }
                                }
                                }
                                frame 1 {
                                }
                                frame 2 {
                                n1817 = Subtract(x=w5580, y=18000.0 ("x")) -> (x-y=w5577:dbl)
                                n1818 = Less Than 0?(x=w5577) -> (x < 0?=w5578:bool)
                                n1819 = case shown="Vrai" w5578 {
                                tunnel: w5577 -> [w5581 w5584]
                                tunnel: [w5581 w5583] -> w5576
                                frame False {
                                }
                                frame True {
                                n1820 = Add(x=w5584, y=86400.0) -> (x+y=w5583:dbl)
                                }
                                }
                                }
                                frame 3, Default {
                                }
                                }
                                n1821 = call "Object_properties.vi"("Target RA"=w5558, "Target DEC"=w5557, "Target Epoch"=w5550, "Sideral Time"=w5551) -> ("NO RA"=w5560:string, "NO DEC"=w5559:string, "NO Epoch"=w5554:dbl, "NO HA"=w5553:dbl, "NO AM"=w5552:dbl)  [unwired: 7 in]
                                n1822 = local write "NO epoch"(w5554) -> ()
                                n1823 = local write "NO AM"(w5552) -> ()
                                n1824 = local write "NO HA"(w5553) -> ()
                                n1825 = local write "N.O. Déc."(w5559) -> ()
                                n1826 = local write "N.O. A.D."(w5560) -> ()
                                }
                                frame #1 {
                                n1827 = call "EXCOM-CMD.vi"("VRN IN"=w5593, "Bool Refnum"=w5587, "Commande #"=12, "Error IN"=w5591) -> ("VRN OUT"=w5589:refnum<visa-resource-name>, "OK Done"=w5588:bool, "Error OUT"=w5590:errorcluster)  [unwired: 9 in]
                                n1828 = case shown="Faux" w5588 {
                                frame False {
                                n1829 = One Button Dialog(message="ATTENTION!!\nLa commande GO a échoué.\nRecommencez ou vérifiez TCS.", button name ("OK")="OK" ("nom du bouton (\"OK\")")) -> ()  [unwired: 1 out]
                                }
                                frame True {
                                }
                                }
                                }
                                }
                                }
                                }
                                }
                                }
                              }
                              frame #2 {
                                n1830 = disable-structure shown="Disabled" {
                                disable-tunnel: w5627 -> [w5628 _]
                                frame Disabled {
                                n1831 = control-ref of="TCS actif"() -> (w5629:refnum<vi>)
                                n1832 = local read "TCS VRN"() -> (w5630:refnum<visa-resource-name>)
                                n1833 = call "EXCOM-CMD.vi"("VRN IN"=w5630, "Bool Refnum"=w5629, "Commande #"=22, "Args"=w5628) -> ()  [unwired: 9 in, 3 out]
                                }
                                frame Enabled {
                                }
                                }
                              }
                            }
                          }
                        }
                      }
                      frame True {
                        w5632 = FALSE
                        n1834 = local write "Zénith"(w5632) -> ()
                        n1835 = local write "Écran"(w5632) -> ()
                        n1836 = local write "Range"(w5632) -> ()
                        n1837 = One Button Dialog(message="ATTENTION!!\nAssurez-vous que l'entraînement sidéral\nest éteint", button name ("OK")="OK" ("nom du bouton (\"OK\")")) -> ()  [unwired: 1 out]
                      }
                    }
                  }
                  frame True {
                    n1838 = local write "Zénith"(w5635) -> ()
                    n1839 = local write "Écran"(w5635) -> ()
                    n1840 = local write "Range"(w5635) -> ()
                    n1841 = One Button Dialog(message="ATTENTION!!\nLe télescope doit être en mode OUEST\npour atteindre cette position ", button name ("OK")="OK" ("nom du bouton (\"OK\")")) -> ()  [unwired: 1 out]
                  }
                }
              }
              event "Origine": Value Change {
                n1842 = event-data() -> ("NewVal"=w5638:bool)  [unwired: 1 in, 4 out]
                n1843 = case shown="Vrai" w5638 {
                  selector: w5638 -> [_ w5639]
                  frame False {
                  }
                  frame True {
                    n1844 = flat-sequence {
                      tunnel: w5639 -> [_]
                      frame #0 {
                        w5641 = 0.0 ("Cible X")
                        n1845 = control-ref of="TERMINAL"() -> (w5645:refnum<vi>)
                        n1846 = control-ref of="Indicateur d'état"() -> (w5644:refnum<vi>)
                        n1847 = local write "Origine"(FALSE ("NeedOrigin")) -> ()
                        n1848 = local write "Cible X"(w5641) -> ()
                        n1849 = local write "Cible Y"(w5641) -> ()
                        n1850 = local write "Cible Z"(w5641) -> ()
                        n1851 = call "TERMINAL.vi"("Indicateur Refnum"=w5644, "Terminal Refnum"=w5645, "Indicateur d'état"="Commande d'origine des tables") -> ()
                        "Origine en cours..." <- TRUE ("Qsleep")
                      }
                      frame #1 {
                        n1852 = flat-sequence {
                          tunnel: [w5658] -> w5647
                          tunnel: [w5654] -> w5646
                          tunnel: w5647 -> [w5660]
                          tunnel: w5646 -> [w5659]
                          frame #0 {
                            # "Si F,F,F -> 0,0,0\nSi F,F,V -> 0,0,1000000"
                            # "Position X, Y, Z après l'initialisation"
                            # "Valeur de vitesse utilisées ..."
                            n1853 = local read "ActiveStages"() -> (w5652:string[])
                            n1854 = local read "Table VRN"() -> (w5648:refnum<visa-resource-name>)
                            n1855 = control-ref of="Exceptions"() -> (w5651:refnum<vi>)
                            n1856 = control-ref of="Table actif"() -> (w5653:refnum<vi>)
                            n1857 = local read "Table Error"() -> (w5655:errorcluster)
                            n1858 = control-ref of="Quit_Origine"() -> (w5650:refnum<vi>)
                            n1859 = call "Newmark-Home.vi"("Table VRN IN"=w5648, "Comm Active"=w5653, "Exceptions"=w5651, "StageTAGs"=w5652, "Velocities"=cluster{"Slow":dbl, "Fast":dbl, "Accel":dbl} {"Slow"=10.0, "Fast"=30000.0, "Accel"=60000.0}, "HomeReverse?"=bool[] [FALSE, FALSE, TRUE], "Error IN"=w5655, "Quit Orgine"=w5650, "EndValues"=i32[] [0, 0, 1000000]) -> ("Table VRN OUT"=w5658:refnum<visa-resource-name>, "Error OUT"=w5654:errorcluster)  [unwired: 5 in]
                          }
                          frame #1 {
                            n1860 = local write "Origine en cours..."(FALSE ("Origine en cours...")) -> ()
                            n1861 = local write "Table VRN"(w5660) -> ()
                            n1862 = local write "Table Error"(w5659) -> ()
                          }
                        }
                        n1863 = while {
                          stop <- w5665 continue-if-true
                          n1864 = Wait (ms)(milliseconds to wait=u32 333) -> ()  [unwired: 1 out]
                          n1865 = local read "enfoncé"() -> (w5662:bool)
                          n1866 = Not(x=w5662) -> (.not. x?=w5663:bool)
                          n1867 = local write "enfoncé"(w5663) -> ()
                          n1868 = local read "Origine en cours..."() -> (w5665:bool)
                        }
                      }
                      frame #2 {
                        w5666 = FALSE ("NeedOrigin")
                        n1869 = local write "NeedOrigin"(w5666) -> ()
                        n1870 = local write "enfoncé"(w5666) -> ()
                        n1871 = property on="Origine" class="Bool (strict)"("Blinking"=FALSE) -> ()  [unwired: 2 in, 2 out]
                      }
                    }
                  }
                }
              }
              event "Centre": Value Change {
                n1872 = event-data() -> ("NewVal"=w5669:bool)  [unwired: 1 in, 4 out]
                n1873 = local write "Centre"(FALSE ("Centre")) -> ()
                n1874 = case shown="Vrai" w5669 {
                  frame False {
                  }
                  frame True {
                    w5672 = TRUE ("CorrectZ")
                    n1875 = control-ref of="TERMINAL"() -> (w5682:refnum<vi>)
                    n1876 = control-ref of="Indicateur d'état"() -> (w5683:refnum<vi>)
                    n1877 = local read "Reference X"() -> (w5675:dbl)
                    n1878 = local read "Reference Y"() -> (w5674:dbl)
                    n1879 = local read "Position Z"() -> (w5673:dbl)
                    n1880 = call "TERMINAL.vi"("Indicateur Refnum"=w5683, "Terminal Refnum"=w5682, "Indicateur d'état"="Commande de déplacement des tables vers le centre") -> ()
                    n1881 = local read "LimXPesto"() -> (w5670:dbl)
                    n1882 = local read "BrasPesto"() -> (w5671:bool)
                    n1883 = local read "Table Error"() -> (w5677:errorcluster)
                    n1884 = local read "Table VRN"() -> (w5681:refnum<visa-resource-name>)
                    n1885 = control-ref of="Table actif"() -> (w5679:refnum<vi>)
                    n1886 = local write "CorrectXY"(w5672) -> ()
                    n1887 = local write "CurvCorrect"(w5672) -> ()
                    n1888 = call "Newmark-GotoAll.vi"("Table VRN IN"=w5681, "BrasPesto"=w5671, "Bool Refnum"=w5679, "LimXPesto"=w5670, "Notify?"=FALSE, "Error IN"=w5677, "Position X"=w5675, "Position Y"=w5674, "Position Z"=w5673) -> ("Table VRN OUT"=w5680:refnum<visa-resource-name>, "Error OUT"=w5676:errorcluster)  [unwired: 5 in]
                    n1889 = local write "Table VRN"(w5680) -> ()
                    n1890 = local write "Table Error"(w5676) -> ()
                    n1891 = local write "Cible X"(w5675) -> ()
                    n1892 = local write "Cible Y"(w5674) -> ()
                    n1893 = local write "Cible Z"(w5673) -> ()
                  }
                }
              }
              event "Alacible": Value Change {
                n1894 = event-data() -> ("NewVal"=w5686:bool)  [unwired: 1 in, 4 out]
                n1895 = case shown="Vrai" w5686 {
                  frame False {
                  }
                  frame True {
                    w5689 = TRUE ("CorrectZ")
                    # "Calcul de la position\nde la sonde en pulse"
                    n1896 = property on="TableXYPos" class="GraphXY (strict)"("Active Cursor"=u32 0) -> ("Cursor.Cursor X"=w5706:dbl, "Cursor.Cursor Y"=w5705:dbl)  [unwired: 2 in, 2 out]
                    n1897 = local read "FieldAstrom"() -> (w5702:T4)
                    n1898 = call "xy2ad.vi"("Y (px)"=w5705, "X (px)"=w5706, "Astrometry"=w5702) -> ("DEC (°)"=w5703:dbl, "RA (°)"=w5704:dbl)  [unwired: 5 in, 2 out]
                    n1899 = local write "CorrectXY"(w5689) -> ()
                    n1900 = local write "CurvCorrect"(w5689) -> ()
                    n1901 = local read "TableAstrom"() -> (w5701:T4)
                    n1902 = call "ad2xy.vi"("DEC"=w5703, "RA"=w5704, "Astrometry"=w5701) -> ("Y"=w5691:dbl, "X"=w5692:dbl)  [unwired: 6 in, 1 out]
                    n1903 = Round To Nearest(number=w5692) -> (nearest integer value=w5688:dbl)
                    n1904 = Round To Nearest(number=w5691) -> (nearest integer value=w5690:dbl)
                    n1905 = Number To Fractional String(number=w5692, precision (6)=i16 0) -> (F-format string=w5697:string)  [unwired: 2 in]
                    n1906 = Number To Fractional String(number=w5691, precision (6)=i16 0) -> (F-format string=w5696:string)  [unwired: 2 in]
                    n1907 = Concatenate Strings("Commande de déplacement des tables vers la cible [" ("Indicateur d'état"), w5697, "," ("Indicateur d'état"), w5696, "]" ("Indicateur d'état")) -> (w5693:string)
                    n1908 = control-ref of="TERMINAL"() -> (w5709:refnum<vi>)
                    n1909 = control-ref of="Indicateur d'état"() -> (w5708:refnum<vi>)
                    n1910 = case shown="Vrai" TRUE {
                      tunnel: w5688 -> [_ w5714]
                      tunnel: w5690 -> [_ w5713]
                      frame False {
                      }
                      frame True {
                        n1911 = local read "Position Z"() -> (w5712:dbl)
                        n1912 = local read "LimXPesto"() -> (w5710:dbl)
                        n1913 = local read "BrasPesto"() -> (w5711:bool)
                        n1914 = local write "Cible X"(w5714) -> ()
                        n1915 = local write "Cible Y"(w5713) -> ()
                        n1916 = local write "Cible Z"(w5712) -> ()
                        n1917 = local read "Table VRN"() -> (w5720:refnum<visa-resource-name>)
                        n1918 = local read "Table Error"() -> (w5718:errorcluster)
                        n1919 = control-ref of="Table actif"() -> (w5715:refnum<vi>)
                        n1920 = call "Newmark-GotoAll.vi"("Table VRN IN"=w5720, "BrasPesto"=w5711, "Bool Refnum"=w5715, "LimXPesto"=w5710, "Notify?"=FALSE, "Error IN"=w5718, "Position X"=w5714, "Position Y"=w5713, "Position Z"=w5712) -> ("Table VRN OUT"=w5719:refnum<visa-resource-name>, "Error OUT"=w5717:errorcluster)  [unwired: 5 in]
                        n1921 = local write "Table VRN"(w5719) -> ()
                        n1922 = local write "Table Error"(w5717) -> ()
                      }
                    }
                    n1923 = call "TERMINAL.vi"("Indicateur Refnum"=w5708, "Terminal Refnum"=w5709, "Indicateur d'état"=w5693) -> ()
                  }
                }
                n1924 = local write "Alacible"(FALSE ("Alacible")) -> ()
              }
              event "Calibration": Value Change {
                w5721 = TRUE ("CorrectZ")
                n1925 = event-data() -> ("NewVal"=w5723:bool)  [unwired: 1 in, 4 out]
                n1926 = local write "CorrectXY"(w5721) -> ()
                n1927 = local write "CurvCorrect"(w5721) -> ()
                n1928 = local write "Calibration"(FALSE ("Calibration")) -> ()
                n1929 = case shown="Vrai" w5723 {
                  frame False {
                  }
                  frame True {
                    n1930 = control-ref of="TERMINAL"() -> (w5735:refnum<vi>)
                    n1931 = control-ref of="Indicateur d'état"() -> (w5736:refnum<vi>)
                    n1932 = call "TERMINAL.vi"("Indicateur Refnum"=w5736, "Terminal Refnum"=w5735, "Indicateur d'état"="Commande de déplacement des tables vers la position de calibration.") -> ()
                    n1933 = local read "BrasPesto"() -> (w5725:bool)
                    n1934 = local read "LimXPesto"() -> (w5724:dbl)
                    n1935 = local read "Table VRN"() -> (w5734:refnum<visa-resource-name>)
                    n1936 = local read "Table Error"() -> (w5732:errorcluster)
                    n1937 = local read "Position Z"() -> (w5726:dbl)
                    n1938 = control-ref of="Table actif"() -> (w5729:refnum<vi>)
                    n1939 = call "Newmark-GotoAll.vi"("Table VRN IN"=w5734, "BrasPesto"=w5725, "Bool Refnum"=w5729, "LimXPesto"=w5724, "Notify?"=FALSE, "Error IN"=w5732, "Position X"="Calibration X", "Position Y"="Calibration Y", "Position Z"=w5726) -> ("Table VRN OUT"=w5733:refnum<visa-resource-name>, "Error OUT"=w5731:errorcluster)  [unwired: 5 in]
                    n1940 = local write "Table VRN"(w5733) -> ()
                    n1941 = local write "Table Error"(w5731) -> ()
                    n1942 = local write "Cible X"("Calibration X") -> ()
                    n1943 = local write "Cible Y"("Calibration Y") -> ()
                    n1944 = local write "Cible Z"(w5726) -> ()
                  }
                }
              }
              event "RangeTable": Value Change {
                n1945 = event-data() -> ("NewVal"=w5739:bool)  [unwired: 1 in, 4 out]
